vi "Image Sinks.vi"() -> ()   [LabVIEW 2020]
uses:
  LabVIEW/g_ar_toolkit.image/ARGB Colour.ctl
  LabVIEW/g_ar_toolkit.common/Image Size (Integer).ctl
  LabVIEW/g_ar_toolkit.image/NewImageARGB.vi
  LabVIEW/g_ar_toolkit.image/CopyImageToPixmapARGBNoMask.vi
  LabVIEW/g_ar_toolkit.image/NewImageARGB.vi/3321fa97-f432-4e1e-8db9-a0df79aed21b.vi
  LabVIEW/g_ar_toolkit.image/ARGB Colour to U32 Pixel Value.vi
  LabVIEW/g_ar_toolkit.image/CopyImageToPixmapARGBNoMask.vi/5c639587-cf36-4d54-93d9-e654c7c24c6e.vi
  LabVIEW/g_ar_toolkit.common/Module Path.vi
  <vilib>/Utility/error.llb/Error Cluster From Error Code.vi
  LabVIEW/g_ar_toolkit.image/g_ar_toolkit.image.lvlib
  LabVIEW/g_ar_toolkit.image/CopyImageToRawMemoryARGB.vi
  LabVIEW/g_ar_toolkit.image/DrawImageToPictureARGB.vi
  LabVIEW/g_ar_toolkit.common/g_ar_toolkit.common.lvlib
panel:
  out "Picture":picture
  out "Picture":picture
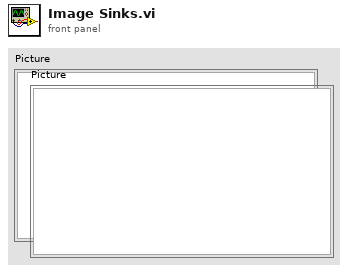
[diagram p1: front panel]
types:
  T1 = typedef "g_ar_toolkit.common.lvlib/Image Size (Integer).ctl" = cluster{"Width":u16, "Height":u16}
  T2 = typedef "g_ar_toolkit.image.lvlib/ARGB Colour.ctl" = cluster{"Alpha":u8, "RGB":u32}
  T3 = typedef "g_ar_toolkit.image.lvlib/ARGB Image.ctl" = refnum<data-value>
  T4 = typedef "imagedata.ctl" = cluster{"image type":i32, "image depth":i32, "image":u8[], "mask":u8[], "colors":u32[], "Rectangle":cluster{"left":i16, "top":i16, "right":i16, "bottom":i16}}
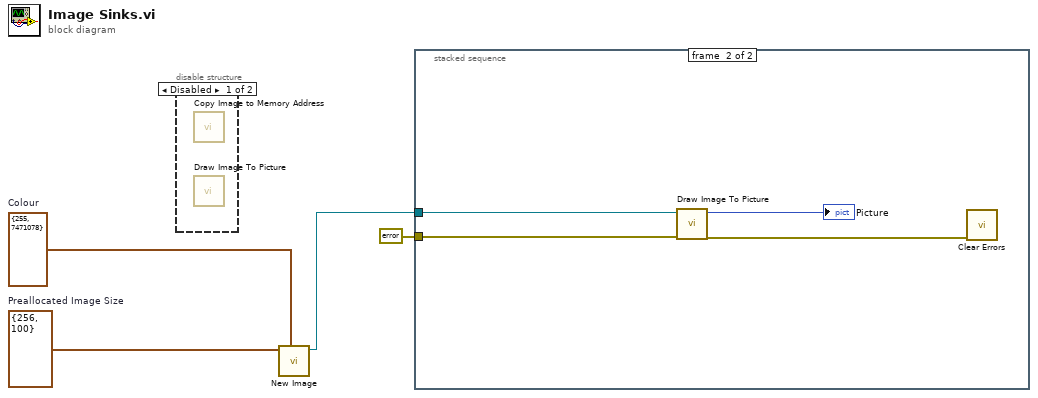
[diagram p0: block diagram]
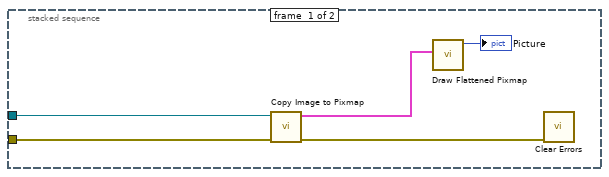
[diagram p2: hidden frame]
diagram:
  w2 = T1 {"Width"=256, "Height"=100}  # Preallocated Image Size
  w3 = T2 {"Alpha"=255, "RGB"=7471078}  # Colour
  n1 = disable-structure shown="Disabled" {
    frame Disabled {
      n2 = call-poly "Copy Image to Memory Address.vi"() -> ()  [unwired: 10 in, 2 out]
      n3 = call-poly "Draw Image To Picture.vi"() -> ()  [unwired: 10 in, 2 out]
    }
    frame Enabled {
    }
  }
  n4 = call-poly "New Image.vi"("Colour (Default: Black)"=w3, "Preallocated Image Size (Default: 0,0)"=w2) -> ("New ARGB Image"=w1:T3)  [unwired: 8 in, 1 out]
  n5 = stacked-sequence {
    tunnel: errorcluster {"status"=FALSE, "code"=0, "source"=""} ("error constant") -> [w8 w13]
    tunnel: w1 -> [w7 w12]
    frame #0 {
      n6 = call-poly "Copy Image to Pixmap.vi"("error in (no error)"=w8, "ARGB Image Source"=w7) -> ("error out"=w5:errorcluster, "Pixmap Image Data"=w9:T4)  [unwired: 8 in]
      n7 = call <vilib>:"Draw Flattened Pixmap.vi"("image data"=w9) -> ("new picture"=→"Picture":picture)  [unwired: 8 in]
      n8 = call <vilib>:"Clear Errors.vi"("error in (no error)"=w5) -> ()  [unwired: 5 in, 2 out]
    }
    frame #1 {
      n9 = call-poly "Draw Image To Picture.vi"("error in (no error)"=w13, "ARGB Image Source"=w12) -> ("error out"=w11:errorcluster, "Picture"=→"Picture":picture)  [unwired: 8 in]
      n10 = call <vilib>:"Clear Errors.vi"("error in (no error)"=w11) -> ()  [unwired: 5 in, 2 out]
    }
  }
